vi "틱을이용한카운터.vi"() -> ()   [LabVIEW 2020]
panel:
  in  "목표시간":dbl
  out "현재시간":dbl
  in  "정지":bool
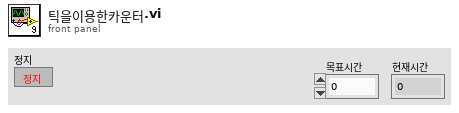
[diagram p1: front panel]
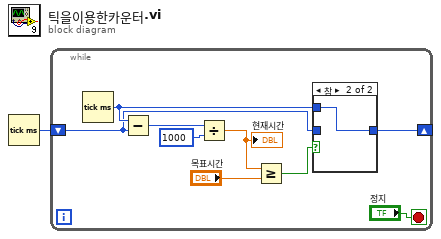
[diagram p0: block diagram]
diagram:
  n1 = Tick Count (ms)() -> (millisecond timer value=w1:u32)
  n2 = while {
    shift-right: [w2] -> _
    shift-left: w1 -> [w4]
    stop <- "정지" stop-if-true
    n3 = Tick Count (ms)() -> (millisecond timer value=w5:u32)
    n4 = Subtract(x=w5, y=w4) -> (x-y=w9:u32)
    n5 = Divide(x=w9, y=u32 1000) -> (x/y=w6:dbl)
    "현재시간" <- w6
    n6 = Greater Or Equal?(x=w6, y="목표시간") -> (x >= y?=w3:bool)
    n7 = case shown="참" w3 {
      tunnel: w5 -> [_ w12]
      tunnel: w4 -> [w11 _]
      tunnel: [w11 w12] -> w2
      frame False {
      }
      frame True {
      }
    }
  }
